vi "ItemSelection_NamesGlobal.vi"() -> ()   [LabVIEW 2014, in "ItemSelection.lvlib"]
uses:
  ItemSelection.lvlib
panel:
  in  "ItemQueueName":string="_VERITECH_LVCM_ITEMSEL_QUEUE_"
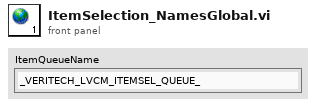
[diagram p1: front panel]
diagram:
